vi "Grab.vi"(0 "ref in":refnum<k7>, 5 "image in":T1, 7 "Timeout":i32, 9 "wait":bool=TRUE, 11 "error in":errorcluster) -> (4 "ref out":refnum<k7>, 6 "image out":T1, 8 "pixel":u32[][](array[numeric]), 10 "index":i32, 15 "error out":errorcluster)   [LabVIEW 2010]
uses:
  <vilib>/vision/Image Controls.llb/IMAQ Image.ctl
  kernel32.dll
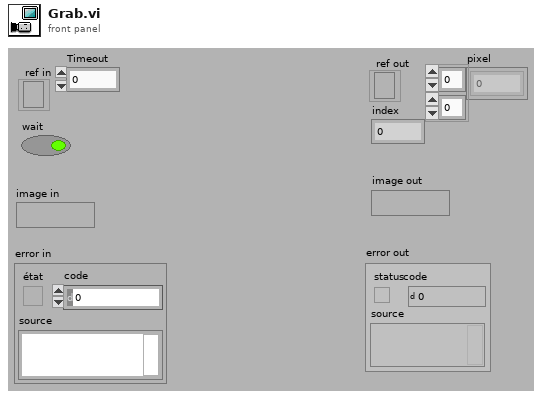
[diagram p1: front panel]
types:
  T1 = typedef "IMAQ Image.ctl" = refnum<image>
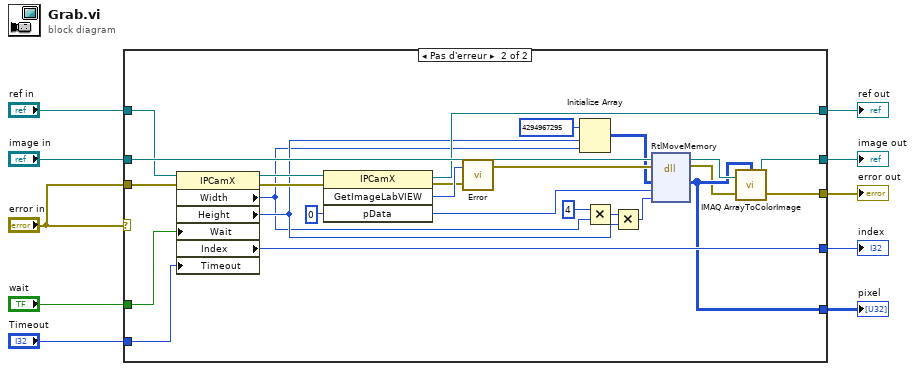
[diagram p0: block diagram]
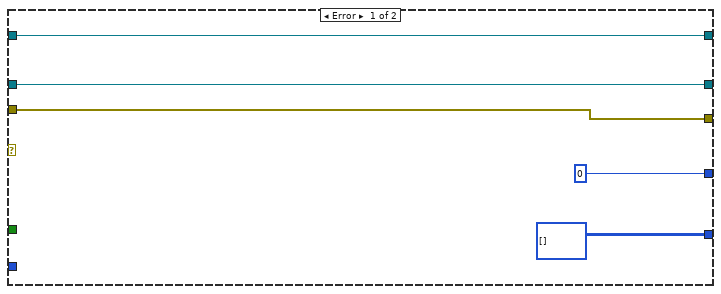
[diagram p2: hidden frame]
diagram:
  n1 = case shown="Pas d'erreur" "error in" {
    tunnel: "image in" -> [w13 w37]
    tunnel: [w13 w31] -> w9
    tunnel: "error in" -> [w11 w35]
    tunnel: "ref in" -> [w12 w36]
    tunnel: [w12 w30] -> w7
    tunnel: "wait" -> [_ w34]
    tunnel: [0 ("Index") w32] -> w5
    tunnel: "Timeout" -> [_ w33]
    tunnel: [u32[][] [] ("Destination") w17] -> w3
    tunnel: [w11 w27] -> w1
    frame Error {
    }
    frame No Error {
      n2 = property class="IPCamX"(reference=w36, error in=w35, "Wait"=w34, "Timeout"=w33) -> (reference out=w40:refnum<k7>, error out=w39:errorcluster, "Width"=w20:i32, "Height"=w23:i32, "Index"=w32:i32)
      n3 = invoke class="IPCamX" method="GetImageLabVIEW"(reference=w40, error in=w39, "pData"=0) -> (reference out=w30:refnum<k7>, error out=w28:errorcluster, "GetImageLabVIEW"=w29:i32, "pData"=w18:i32)  [unwired: 1 in]
      n4 = call "Error.vi"("error in"=w28, "code"=w29) -> ("error out"=w26:errorcluster)
      n5 = Initialize Array(u32 4294967295, w23, w20) -> (w19:u32[][])
      n6 = Multiply(x=4 ("y"), y=w20) -> (x*y=w22:i32)
      n7 = Multiply(x=w22, y=w23) -> (x*y=w24:u32)
      n8 = dll-call lib="kernel32.dll" fn="RtlMoveMemory"(error in=w26, "Destination"=w19, "Source"=w18, "Size"=w24) -> (error out=w16:errorcluster, "Destination"=w17:u32[][])  [unwired: 5 in, 1 out]
      n9 = call "IMAQ ArrayToColorImage"("Image Pixels (U32)"=w17, "Image"=w37, "error in (no error)"=w16) -> ("Image Out"=w31:T1, "error out"=w27:errorcluster)  [unwired: 2 in]
    }
  }
  "image out" <- w9
  "error out" <- w1
  "ref out" <- w7
  "index" <- w5
  "pixel" <- w3
